vi "satrecGenerator.vi"(4 "parametres_TLE":cdb[][](array[numeric])) -> (0 "jddecimal":cdb, 1 "jd":cdb, 2 "satrec":T1)   [LabVIEW 2015]
uses:
  <vilib>/imath/engines/lvmath2/RunTimeEngine/Managers/WorkSpace/UID Generator.vi
  <vilib>/imath/engines/lvmath2/RunTimeEngine/RunTimeType/NIMS_RunTimeType_From StrictType (excl LVString).vi
  <instcachedir>/0/NIMS_RunTimeType_From StrictType (excl LVString)_EB1C38A9BC5048DA9ABDA8F781E54D21.lvgen/NIMS_RunTimeType_From StrictType (excl LVString)_EB1C38A9BC5048DA9ABDA8F781E54D21_032.vi
  <instcachedir>/0/NIMS_RunTimeType_From StrictType (excl LVString)_EB1C38A9BC5048DA9ABDA8F781E54D21.lvgen/NIMS_RunTimeType_From StrictType (excl LVString)_EB1C38A9BC5048DA9ABDA8F781E54D21_031.vi
  <vilib>/imath/engines/lvmath/Plug In/_Char/NIMS_CH_String CV to Character 2D.vi
  <instcachedir>/0/NIMS_CH_String CV to Character 2D_EC8CCB3F0D074D66A728E5B1D55F815A.lvgen/NIMS_CH_String CV to Character 2D_EC8CCB3F0D074D66A728E5B1D55F815A_000.vi
  <instcachedir>/0/NIMS_RunTimeType_From StrictType (excl LVString)_EB1C38A9BC5048DA9ABDA8F781E54D21.lvgen/NIMS_RunTimeType_From StrictType (excl LVString)_EB1C38A9BC5048DA9ABDA8F781E54D21_001.vi
  <vilib>/imath/engines/lvmath2/RunTimeEngine/Struct/NIMS_StructSetField.vi
  <vilib>/imath/engines/lvmath2/RunTimeEngine/IndexRead/NIMS M(S).vi
  <instcachedir>/0/NIMS M(S)_B826C018497E4940AE96BD27B540B6FB.lvgen/NIMS M(S)_B826C018497E4940AE96BD27B540B6FB_004.vi
  <instcachedir>/0/NIMS_RunTimeType_From StrictType (excl LVString)_EB1C38A9BC5048DA9ABDA8F781E54D21.lvgen/NIMS_RunTimeType_From StrictType (excl LVString)_EB1C38A9BC5048DA9ABDA8F781E54D21_030.vi
  <vilib>/imath/engines/lvmath2/RunTimeEngine/Struct/NIMS_StructGetField.vi
  <vilib>/imath/engines/lvmath2/RunTimeEngine/RunTimeType/NIMS_RunTimeType_To Numeric.vi
  <instcachedir>/0/NIMS_RunTimeType_To Numeric_B134FEC7BFC54ED5998F4CFD2EE98288.lvgen/NIMS_RunTimeType_To Numeric_B134FEC7BFC54ED5998F4CFD2EE98288_008.vi
  <instcachedir>/0/NIMS_RunTimeType_From StrictType (excl LVString)_EB1C38A9BC5048DA9ABDA8F781E54D21.lvgen/NIMS_RunTimeType_From StrictType (excl LVString)_EB1C38A9BC5048DA9ABDA8F781E54D21_000.vi
  <instcachedir>/0/NIMS_RunTimeType_To Numeric_B134FEC7BFC54ED5998F4CFD2EE98288.lvgen/NIMS_RunTimeType_To Numeric_B134FEC7BFC54ED5998F4CFD2EE98288_007.vi
  <instcachedir>/0/NIMS_RunTimeType_To Numeric_B134FEC7BFC54ED5998F4CFD2EE98288.lvgen/NIMS_RunTimeType_To Numeric_B134FEC7BFC54ED5998F4CFD2EE98288_009.vi
  <instcachedir>/0/NIMS_RunTimeType_From StrictType (excl LVString)_EB1C38A9BC5048DA9ABDA8F781E54D21.lvgen/NIMS_RunTimeType_From StrictType (excl LVString)_EB1C38A9BC5048DA9ABDA8F781E54D21_003.vi
  <vilib>/imathl/engines/lvmath/Functions/Error Handling/Create Error.vi
  <vilib>/imath/engines/lvmath2/RunTimeEngine/LocalVariableDefStatement/MC_LocalVariableDefStatement_Display.vi
  <vilib>/imath/engines/lvmath2/RunTimeEngine/ArithmeticOperatorToken/NIMS_ArithmeticOperator_power(S).vi
  <instcachedir>/0/NIMS_ArithmeticOperator_power(S)_DFB67823F1414E5097C86E39787D8CA8.lvgen/NIMS_ArithmeticOperator_power(S)_DFB67823F1414E5097C86E39787D8CA8_015.vi
  <instcachedir>/0/NIMS_ArithmeticOperator_power(S)_DFB67823F1414E5097C86E39787D8CA8.lvgen/NIMS_ArithmeticOperator_power(S)_DFB67823F1414E5097C86E39787D8CA8_009.vi
  <vilib>/imath/engines/lvmath/Plug In/_Char/RunTimeType/NIMS_CH_RunTimeType_To Character 2D.vi
  <vilib>/imath/engines/lvmath/Plug In/_Char/NIMS_CH_Character 2D to String 1D.vi
  <vilib>/imath/engines/lvmath2/RunTimeEngine/RangeToken/NIMS_Range_R2 - Integer.vi
  <instcachedir>/0/NIMS_Range_R2 - Integer_396D5D4FB869421F9245109A0975AD54.lvgen/NIMS_Range_R2 - Integer_396D5D4FB869421F9245109A0975AD54_000.vi
  <vilib>/imath/engines/lvmath2/RunTimeEngine/CommandStatement/MC_CommandStatement_break.vi
  <vilib>/imath/engines/lvmath2/RunTimeEngine/VariableToken/NIMS_VariableToken_CondDefinedDefinedByReplace.vi
  <instcachedir>/0/NIMS_VariableToken_CondDefinedDefinedByReplace_D162CFFC24174562A9FEA619A91E1A56.lvgen/NIMS_VariableToken_CondDefinedDefinedByReplace_D162CFFC24174562A9FEA619A91E1A56_002.vi
  <vilib>/imath/engines/lvmath2/RunTimeEngine/IndexReplace/NIMS V(S)=S.vi
  <instcachedir>/0/NIMS V(S)=S_9916D32195284AEB9D40BA9A64F3B0C5.lvgen/NIMS V(S)=S_9916D32195284AEB9D40BA9A64F3B0C5_004.vi
  <vilib>/imath/engines/lvmath2/RunTimeSupport/NIMS_Complex To Real.vi
  <instcachedir>/0/NIMS_Complex To Real_01315F44AA8B4CE79FEF95AE999DC25E.lvgen/NIMS_Complex To Real_01315F44AA8B4CE79FEF95AE999DC25E_001.vi
  <vilib>/imath/engines/lvmath2/RunTimeEngine/BuiltInFunctions/rem/NIMS_rem_no checks.vi
  <instcachedir>/0/NIMS_rem_no checks_948DC4F3B45040069021B8F54D02F312.lvgen/NIMS_rem_no checks_948DC4F3B45040069021B8F54D02F312_000.vi
  <vilib>/imath/engines/lvmath2/RunTimeEngine/VariableToken/NIMS_VariableToken_CondDefined.vi
  <instcachedir>/0/NIMS_VariableToken_CondDefined_FE30D0A1BFB24F098D41DEBABFE96BE1.lvgen/NIMS_VariableToken_CondDefined_FE30D0A1BFB24F098D41DEBABFE96BE1_004.vi
  <vilib>/imath/engines/lvmath2/RunTimeEngine/IndexRead/NIMS V(S).vi
  <instcachedir>/0/NIMS V(S)_0488751826AF41519A22953C041130DC.lvgen/NIMS V(S)_0488751826AF41519A22953C041130DC_002.vi
  <vilib>/imath/engines/lvmath2/RunTimeEngine/ErrorHandling/NIMS_Create Error From Enums.vi
  <vilib>/imath/engines/lvmath2/RunTimeEngine/CommandStatement/NIMS_CommandStatement_MaskErr.vi
  <vilib>/imath/engines/lvmath2/RunTimeEngine/BuiltInFunctions/fix/NIMS_fix(CDB-S).vi
  <vilib>/imath/engines/lvmath2/RunTimeEngine/Managers/SymbolTable/Clear UID.vi
  <vilib>/imath/engines/lvmath2/RunTimeEngine/NodeEndStatement/NIMS_NodeEndStatement_Output.vi
  <instcachedir>/0/NIMS_NodeEndStatement_Output_53EC0D466D134D7ABD903AC30B43404B.lvgen/NIMS_NodeEndStatement_Output_53EC0D466D134D7ABD903AC30B43404B_013.vi
  <instcachedir>/0/NIMS_NodeEndStatement_Output_53EC0D466D134D7ABD903AC30B43404B.lvgen/NIMS_NodeEndStatement_Output_53EC0D466D134D7ABD903AC30B43404B_009.vi
  <instcachedir>/0/NIMS_NodeEndStatement_Output_53EC0D466D134D7ABD903AC30B43404B.lvgen/NIMS_NodeEndStatement_Output_53EC0D466D134D7ABD903AC30B43404B_001.vi
  <instcachedir>/0/NIMS_NodeEndStatement_Output_53EC0D466D134D7ABD903AC30B43404B.lvgen/NIMS_NodeEndStatement_Output_53EC0D466D134D7ABD903AC30B43404B_012.vi
  <vilib>/imath/engines/lvmath2/RunTimeEngine/ErrorHandling/NIMS_Finalize Error.vi
  <vilib>/imath/engines/lvmath2/RunTimeEngine/Managers/SymbolTable/NIMS_WorkSpace.lvlib
panel:
  in  "input cluster":T2
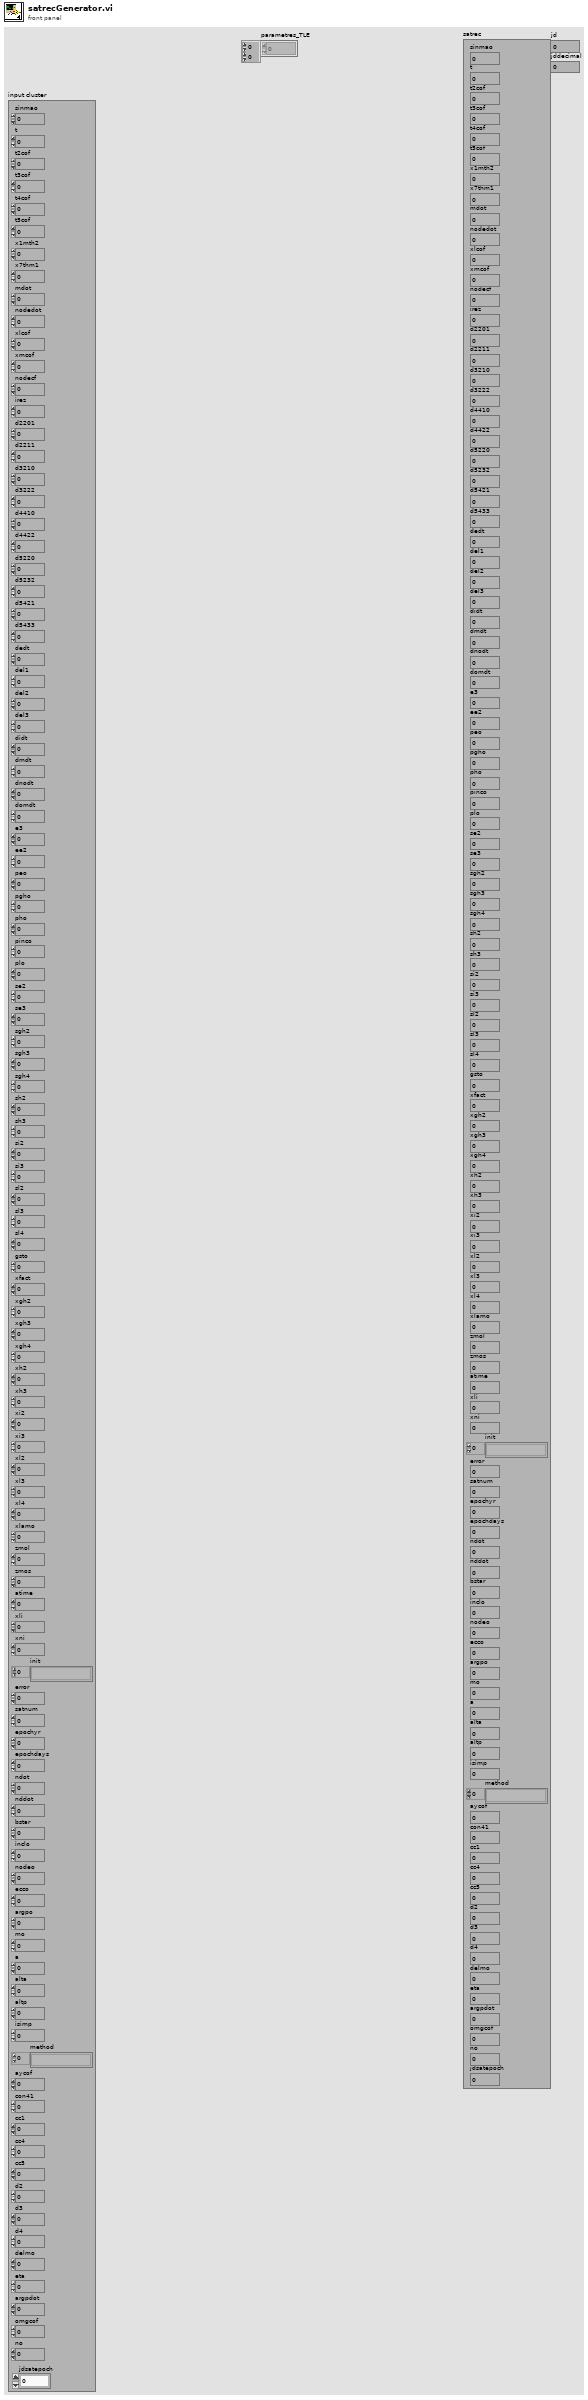
[diagram p1: front panel]
types:
  T1 = cluster{"sinmao":sgl, "t":sgl, "t2cof":sgl, "t3cof":sgl, "t4cof":sgl, "t5cof":sgl, "x1mth2":sgl, "x7thm1":sgl, "mdot":sgl, "nodedot":sgl, "xlcof":sgl, "xmcof":sgl, "nodecf":sgl, "irez":sgl, "d2201":sgl, "d2211":sgl, "d3210":sgl, "d3222":sgl, "d4410":sgl, "d4422":sgl, "d5220":sgl, "d5232":sgl, "d5421":sgl, "d5433":sgl, "dedt":sgl, "del1":sgl, "del2":sgl, "del3":sgl, "didt":sgl, "dmdt":sgl, "dnodt":sgl, "domdt":sgl, "e3":sgl, "ee2":sgl, "peo":sgl, "pgho":sgl, "pho":sgl, "pinco":sgl, "plo":sgl, "se2":sgl, "se3":sgl, "sgh2":sgl, "sgh3":sgl, "sgh4":sgl, "sh2":sgl, "sh3":sgl, "si2":sgl, "si3":sgl, "sl2":sgl, "sl3":sgl, "sl4":sgl, "gsto":sgl, "xfact":sgl, "xgh2":sgl, "xgh3":sgl, "xgh4":sgl, "xh2":sgl, "xh3":sgl, "xi2":sgl, "xi3":sgl, "xl2":sgl, "xl3":sgl, "xl4":sgl, "xlamo":sgl, "zmol":sgl, "zmos":sgl, "atime":sgl, "xli":sgl, "xni":sgl, "init":string[], "error":sgl, "satnum":cdb, "epochyr":cdb, "epochdays":cdb, "ndot":cdb, "nddot":cdb, "bstar":cdb, "inclo":cdb, "nodeo":cdb, "ecco":cdb, "argpo":cdb, "mo":cdb, "a":cdb, "alta":cdb, "altp":cdb, "isimp":sgl, "method":string[], "aycof":sgl, "con41":sgl, "cc1":sgl, "cc4":sgl, "cc5":sgl, "d2":sgl, "d3":sgl, "d4":sgl, "delmo":sgl, "eta":sgl, "argpdot":sgl, "omgcof":sgl, "no":cdb, "jdsatepoch":dbl}
  T2 = cluster{"sinmao":sgl, "t":sgl, "t2cof":sgl, "t3cof":sgl, "t4cof":sgl, "t5cof":sgl, "x1mth2":sgl, "x7thm1":sgl, "mdot":sgl, "nodedot":sgl, "xlcof":sgl, "xmcof":sgl, "nodecf":sgl, "irez":sgl, "d2201":sgl, "d2211":sgl, "d3210":sgl, "d3222":sgl, "d4410":sgl, "d4422":sgl, "d5220":sgl, "d5232":sgl, "d5421":sgl, "d5433":sgl, "dedt":sgl, "del1":sgl, "del2":sgl, "del3":sgl, "didt":sgl, "dmdt":sgl, "dnodt":sgl, "domdt":sgl, "e3":sgl, "ee2":sgl, "peo":sgl, "pgho":sgl, "pho":sgl, "pinco":sgl, "plo":sgl, "se2":sgl, "se3":sgl, "sgh2":sgl, "sgh3":sgl, "sgh4":sgl, "sh2":sgl, "sh3":sgl, "si2":sgl, "si3":sgl, "sl2":sgl, "sl3":sgl, "sl4":sgl, "gsto":sgl, "xfact":sgl, "xgh2":sgl, "xgh3":sgl, "xgh4":sgl, "xh2":sgl, "xh3":sgl, "xi2":sgl, "xi3":sgl, "xl2":sgl, "xl3":sgl, "xl4":sgl, "xlamo":sgl, "zmol":sgl, "zmos":sgl, "atime":sgl, "xli":sgl, "xni":sgl, "init":string[], "error":sgl, "satnum":sgl, "epochyr":sgl, "epochdays":dbl, "ndot":sgl, "nddot":sgl, "bstar":sgl, "inclo":sgl, "nodeo":sgl, "ecco":sgl, "argpo":sgl, "mo":sgl, "a":sgl, "alta":sgl, "altp":sgl, "isimp":sgl, "method":string[], "aycof":sgl, "con41":sgl, "cc1":sgl, "cc4":sgl, "cc5":sgl, "d2":sgl, "d3":sgl, "d4":sgl, "delmo":sgl, "eta":sgl, "argpdot":sgl, "omgcof":sgl, "no":sgl, "jdsatepoch":dbl}
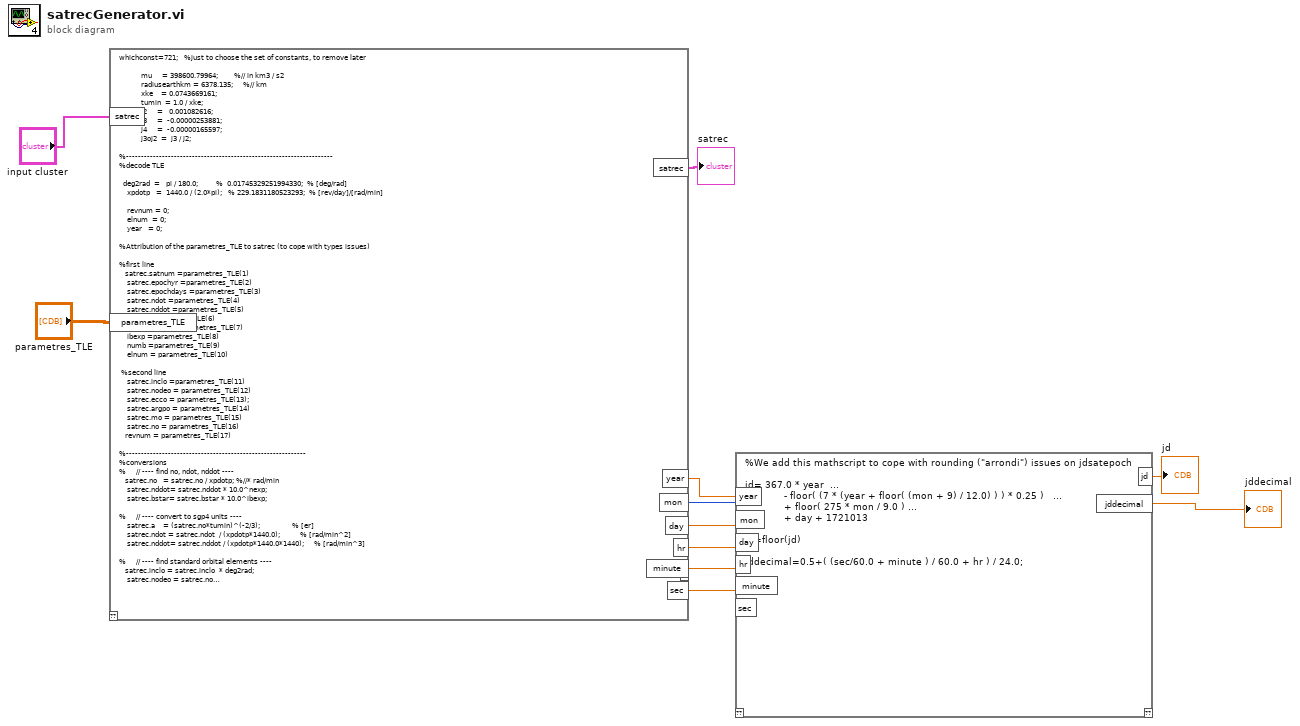
[diagram p0: block diagram]
diagram:
  n1 = mathscript code="whichconst=721;   %just to choose the set of constants, to remove later\n\n           mu     = 398600.79964;        %// in km3 / s2\n           radiusearthkm = 6378.135;     %// km\n           xke    = 0.0743669161;\n           tumin  = 1.0 / xke;\n           j2     =   0.001082616;\n           j3     =  -0.00000253881;\n           j4     =  -0.00000165597;\n           j3oj2  =  j3 / j2;\n\n%---------------------------------------------------------------------\n%decode TLE\n\n  deg2rad  =   pi / 180.0;         %  0.01745329251994330;  % [deg/rad]\n    xpdotp   =  1440.0 / (2.0*pi);   % 229.1831180523293;  % [rev/day]/[rad/min]  \n\n    revnum = 0; \n    elnum  = 0;\n    year   = 0; \n  \n%Attribution of the parametres_TLE to satrec (to cope with types issues)\n\n%first line\n   satrec.satnum =parametres_TLE(1)\n    satrec.epochyr =parametres_TLE(2)\n    satrec.epochdays =parametres_TLE(3)\n    satrec.ndot =parametres_TLE(4)\n    satrec.nddot =parametres_TLE(5)\n   nexp =parametres_TLE(6)\n    satrec.bstar =parametres_TLE(7)\n    ibexp =parametres_TLE(8)\n    numb =parametres_TLE(9)\n    elnum = parametres_TLE(10)\n    \n %second line\n    satrec.inclo =parametres_TLE(11)\n    satrec.nodeo = parametres_TLE(12)\n    satrec.ecco = parametres_TLE(13);\n    satrec.argpo = parametres_TLE(14)\n    satrec.mo = parametres_TLE(15)\n    satrec.no = parametres_TLE(16)\n   revnum = parametres_TLE(17)\n\n%------------------------------------------------------------\n%conversions\n%     // ---- find no, ndot, nddot ----\n   satrec.no   = satrec.no / xpdotp; %//* rad/min\n    satrec.nddot= satrec.nddot * 10.0^nexp;\n    satrec.bstar= satrec.bstar * 10.0^ibexp;\n\n%     // ---- convert to sgp4 units ----\n    satrec.a    = (satrec.no*tumin)^(-2/3);                % [er]\n    satrec.ndot = satrec.ndot  / (xpdotp*1440.0);          % [rad/min^2]\n    satrec.nddot= satrec.nddot / (xpdotp*1440.0*1440);     % [rad/min^3]\n\n%     // ---- find standard orbital elements ----\n   satrec.inclo = satrec.inclo  * deg2rad;\n    satrec.nodeo = satrec.nodeo * deg2rad;\n    satrec.argpo = satrec.argpo  * deg2rad;\n    satrec.mo    = satrec.mo     *deg2rad;\n\n    satrec.alta = satrec.a*(1.0 + satrec.ecco) - 1.0;\n    satrec.altp = satrec.a*(1.0 - satrec.ecco) - 1.0;\n\n%     // ----------------------------------------------------------------\n%     // find sgp4epoch time of element set\n%     // remember that sgp4 uses units of days from 0 jan 1950 (sgp4epoch)\n%     // and minutes from the epoch (time)\n%     // --------------------------------------------------------------\n\n%     // ------------- temp fix for years from 1957-2056 ----------------\n%     // ------ correct fix will occur when year is 4-digit in 2le ------\n     if (satrec.epochyr < 57)\n         year= satrec.epochyr + 2000;\n       else\n         year= satrec.epochyr + 1900;\n    end;\n\n%--------------------------------------------------------------------------------\n%Calculation of month, day, hour, minute, second\n\n % --------------- set up array of days in month  --------------\n        for i= 1 : 12\n            lmonth(i) = 31;\n            if i == 2\n                lmonth(i)= 28;\n              end;\n            if i == 4 | i == 6 | i == 9 | i == 11\n                lmonth(i)= 30;\n              end;\n        end\n\n        dayofyr= floor(satrec.epochdays );\n\n        % ----------------- find month and day of month ---------------\n        if rem(year-1900,4) == 0\n            lmonth(2)= 29;\n          end\n\n        i= 1;\n        inttemp= 0;\n        while ( dayofyr > inttemp + lmonth(i) ) & ( i < 12 )\n            inttemp= inttemp + lmonth(i);\n            i= i+1;\n          end\n\n        mon= i;\n        day= dayofyr - inttemp;\n\n        % ----------------- find hours minutes and seconds ------------\n        temp= (satrec.epochdays - dayofyr )*24.0;\n        hr  = fix( temp );\n        temp= (temp-hr) * 60.0;\n        minute = fix( temp );\n        sec = (temp-minute) * 60.0;\n % --------------- set up array of days in month  --------------\n        for i= 1 : 12\n            lmonth(i) = 31;\n            if i == 2\n                lmonth(i)= 28;\n              end;\n            if i == 4 | i == 6 | i == 9 | i == 11\n                lmonth(i)= 30;\n              end;\n        end\n\n        dayofyr= floor(satrec.epochdays );\n\n        % ----------------- find month and day of month ---------------\n        if rem(year-1900,4) == 0\n            lmonth(2)= 29;\n          end\n\n        i= 1;\n        inttemp= 0;\n        while ( dayofyr > inttemp + lmonth(i) ) & ( i < 12 )\n            inttemp= inttemp + lmonth(i);\n            i= i+1;\n          end\n\n        mon= i;\n        day= dayofyr - inttemp;\n\n        % ----------------- find hours minutes and seconds ------------\n        temp= (satrec.epochdays - dayofyr )*24.0;\n        hr  = fix( temp );\n        temp= (temp-hr) * 60.0;\n        minute = fix( temp );\n        sec = (temp-minute) * 60.0;\n\n\n\n\n %satrec.jdsatepoch= jday(year,mon,day,hr,minute,sec );"("satrec"="input cluster", "parametres_TLE"="parametres_TLE") -> ("mon"=w9:i32, "day"=w8:dbl, "hr"=w7:cdb, "minute"=w6:cdb, "sec"=w5:cdb, "year"=w11:cdb, "satrec"=→"satrec":T1)  [unwired: 1 in, 1 out]
  n2 = mathscript code="%We add this mathscript to cope with rounding (\"arrondi\") issues on jdsatepoch\n\njd= 367.0 * year  ...\n             - floor( (7 * (year + floor( (mon + 9) / 12.0) ) ) * 0.25 )   ...\n             + floor( 275 * mon / 9.0 ) ...\n             + day + 1721013  \n             \njd=floor(jd)\n\njddecimal=0.5+( (sec/60.0 + minute ) / 60.0 + hr ) / 24.0;"("mon"=w9, "day"=w8, "hr"=w7, "minute"=w6, "sec"=w5, "year"=w11) -> ("jd"=→"jd":cdb, "jddecimal"=→"jddecimal":cdb)  [unwired: 1 in, 1 out]
